vi "lab2.vi"   [LabVIEW 2018]
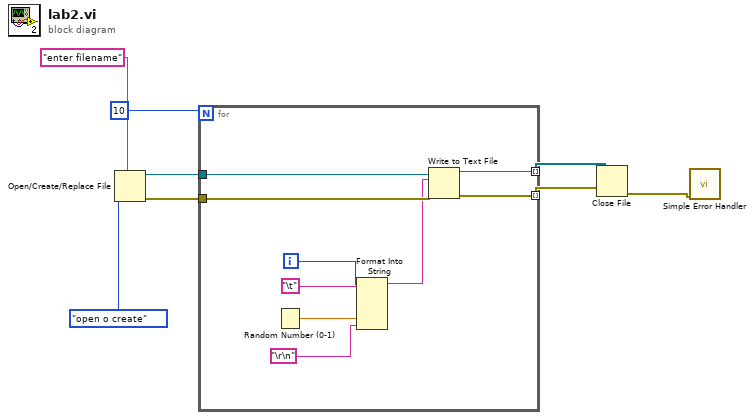
[diagram p0: block diagram]
diagram:
  n1 = Open/Create/Replace File(prompt="enter filename", access (0:read/write)=enum16{"open o create"}."open o create") -> (refnum out=w7:refnum<file>, error out=w6:errorcluster)  [unwired: 4 in, 1 out]
  n2 = for {
    N: 10 -> [_]
    tunnel: w7 -> [w13]
    tunnel: w6 -> [w12]
    tunnel: [w10] -> w5 mode=indexing
    tunnel: [w9] -> w4 mode=indexing
    i -> [w14]
    n3 = Random Number (0-1)() -> (number: 0 to 1=w16:dbl)
    n4 = Format Into String(w14, "\t", w16, "\r\n") -> (resulting string=w11:string)  [unwired: 3 in, 1 out]
    n5 = Write to Text File(file (use dialog)=w13, text=w11, error in=w12) -> (refnum out=w9:refnum<file>, error out=w10:errorcluster)  [unwired: 1 in, 1 out]
  }
  n6 = Close File(refnum=w4, error in=w5) -> (error out=w1:errorcluster)  [unwired: 1 out]
  n7 = call <vilib>:"Simple Error Handler.vi"("error in (no error)"=w1) -> ()  [unwired: 4 in, 5 out]
